vi "Write.vi"(8 "error in (no error)":errorcluster, 10 "Value":T1=variant(string ""), 11 "Double Float.lvclass_340760 in":refnum<class "Var_Variant.lvclass">) -> (0 "error out":errorcluster, 3 "Double Float.lvclass_340760 out":refnum<class "Var_Variant.lvclass">)   [LabVIEW 2021, in "Var_Variant.lvclass"]
uses:
  Var_Variant.lvclass
  Type.ctl
  Var_Variant.lvclass/Var_Variant.ctl
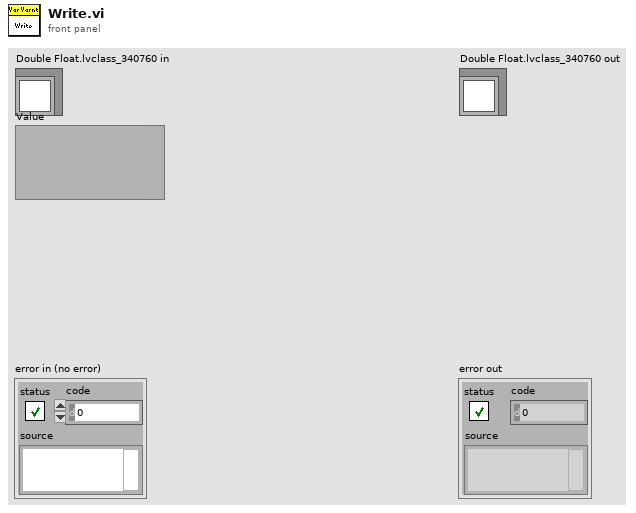
[diagram p1: front panel]
types:
  T1 = typedef "Var_Variant.lvclass/Type.ctl" = variant
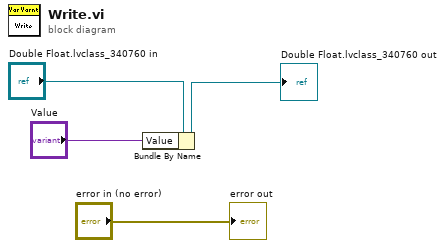
[diagram p0: block diagram]
diagram:
  n1 = Bundle By Name(cluster="Double Float.lvclass_340760 in", "Value"="Value") -> (→"Double Float.lvclass_340760 out":refnum<class "Var_Variant.lvclass">)
  "error out" <- "error in (no error)"
